vi "GenerateCmd.vi"(7 "Cmd":T1, 8 "error in":errorcluster, 10 "exp#":string, 11 "lang.font.exp":string) -> (0 "error Out":errorcluster, 3 "CMD":string)   [LabVIEW 2019]
uses:
  Controls/cmd.ctl
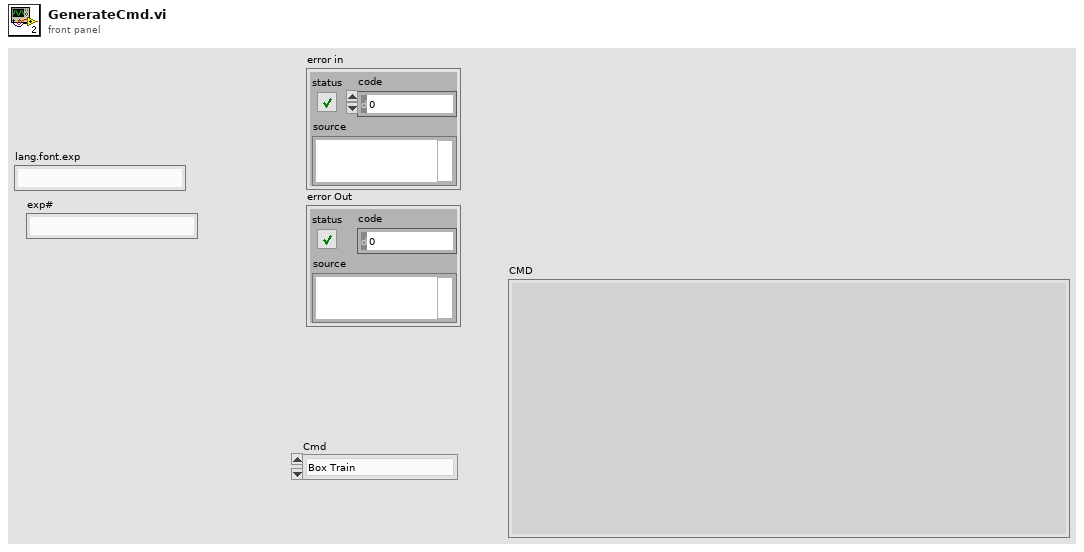
[diagram p1: front panel]
types:
  T1 = typedef "cmd.ctl" = enum16{"Box Train", "unicharset", "ShapeTable", "mftraining1", "mftraining2", "cntraining", "rename", "move files", "combine"}
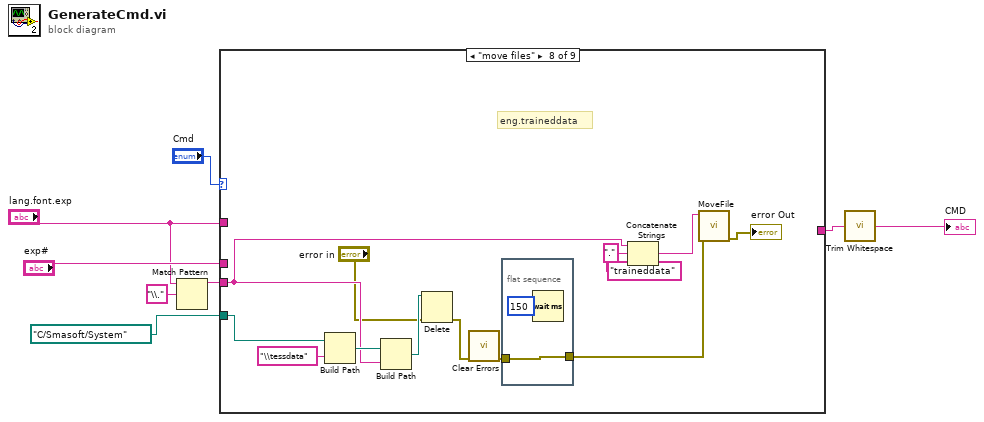
[diagram p0: block diagram]
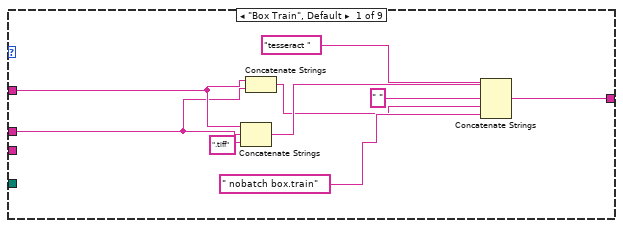
[diagram p2: hidden frame]
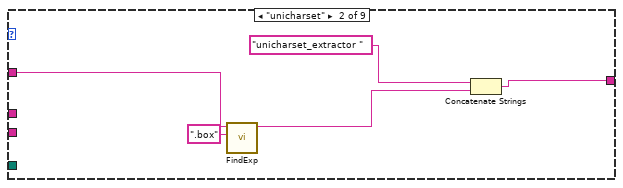
[diagram p3: hidden frame]
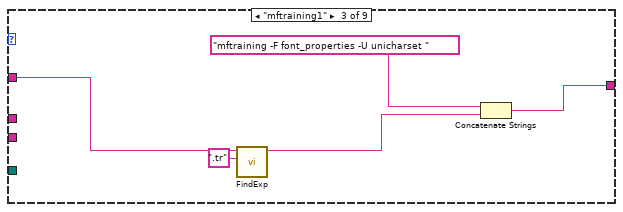
[diagram p4: hidden frame]
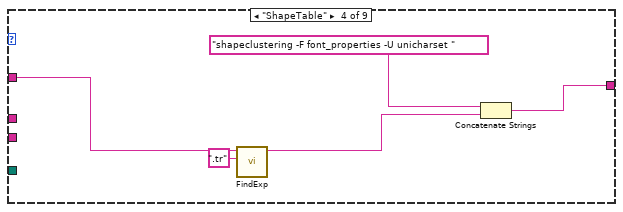
[diagram p5: hidden frame]
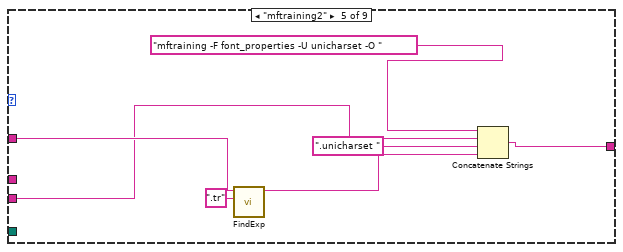
[diagram p6: hidden frame]
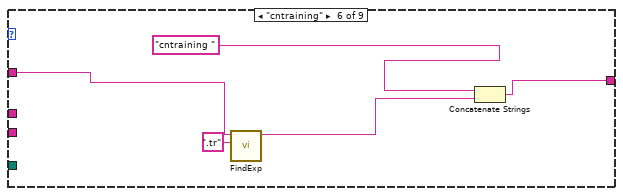
[diagram p7: hidden frame]
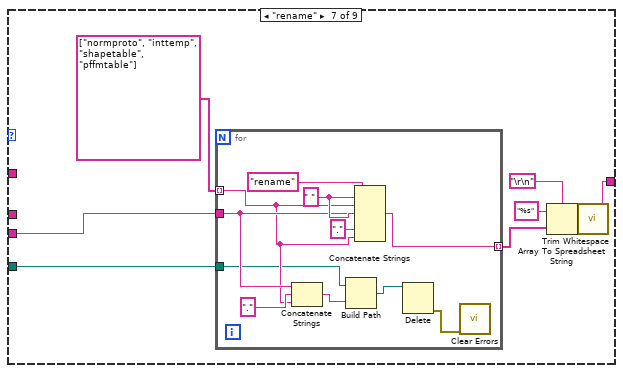
[diagram p8: hidden frame]
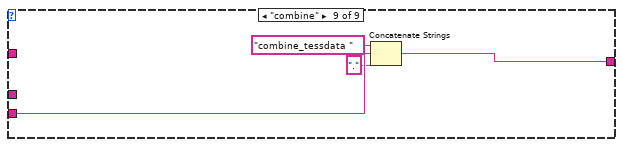
[diagram p9: hidden frame]
diagram:
  n1 = Match Pattern(string="lang.font.exp", regular expression="\\.") -> (before substring=w4:string)  [unwired: 1 in, 3 out]
  n2 = case shown="\"move files\"" "Cmd" {
    tunnel: "lang.font.exp" -> [w11 w20 w25 w30 w37 w41 _ _ _]
    tunnel: [w16 w22 w23 w28 w36 w40 w46 _ w79] -> w3
    tunnel: "exp#" -> [w10 _ _ _ _ _ _ _ _]
    tunnel: w4 -> [_ _ _ _ w34 _ w52 w69 w81]
    tunnel: path "C:/Smasoft/System" ("base path") -> [_ _ _ _ _ _ w45 w72 _]
    frame "Box Train", Default {
      n3 = Concatenate Strings(w11, w10, ".tiff" ("lang.font.exp")) -> (w15:string)
      n4 = Concatenate Strings(w11, w10) -> (w9:string)
      n5 = Concatenate Strings("tesseract ", w15, " " ("string"), w9, " nobatch box.train" ("string")) -> (w16:string)
    }
    frame "unicharset" {
      n6 = call "FindExp.vi"("extension name"=".box", "lang_font.exp"=w20) -> ("spreadsheet string"=w19:string)  [unwired: 9 in]
      n7 = Concatenate Strings("unicharset_extractor ", w19) -> (w22:string)
    }
    frame "mftraining1" {
      n8 = call "FindExp.vi"("extension name"=".tr", "lang_font.exp"=w25) -> ("spreadsheet string"=w26:string)  [unwired: 9 in]
      n9 = Concatenate Strings("mftraining -F font_properties -U unicharset ", w26) -> (w23:string)
    }
    frame "ShapeTable" {
      n10 = call "FindExp.vi"("extension name"=".tr", "lang_font.exp"=w30) -> ("spreadsheet string"=w31:string)  [unwired: 9 in]
      n11 = Concatenate Strings("shapeclustering -F font_properties -U unicharset ", w31) -> (w28:string)
    }
    frame "mftraining2" {
      n12 = call "FindExp.vi"("extension name"=".tr", "lang_font.exp"=w37) -> ("spreadsheet string"=w38:string)  [unwired: 9 in]
      n13 = Concatenate Strings("mftraining -F font_properties -U unicharset -O ", w34, ".unicharset " ("string"), w38) -> (w36:string)
    }
    frame "cntraining" {
      n14 = call "FindExp.vi"("extension name"=".tr", "lang_font.exp"=w41) -> ("spreadsheet string"=w42:string)  [unwired: 9 in]
      n15 = Concatenate Strings("cntraining ", w42) -> (w40:string)
    }
    frame "rename" {
      n16 = for {
        tunnel: string[] ["normproto", "inttemp", "shapetable", "pffmtable"] ("File name") -> [w57] mode=indexing
        tunnel: w52 -> [w59]
        tunnel: [w60] -> w50 mode=indexing
        tunnel: w45 -> [w55]
        w62 = " " ("string")
        n17 = Concatenate Strings(w59, "." ("string"), w57) -> (w56:string)
        n18 = Build Path(base path=w55, name or relative path=w56) -> (appended path=w54:path)
        n19 = Concatenate Strings("rename" ("string"), w62, w57, w62, w59, "." ("string"), w57) -> (w60:string)
        n20 = Delete(path (use dialog)=w54) -> (error out=w53:errorcluster)  [unwired: 4 in, 2 out]
        n21 = call <vilib>:"Clear Errors.vi"("error in (no error)"=w53) -> ()  [unwired: 5 in, 2 out]
      }
      n22 = Array To Spreadsheet String(delimiter (Tab)="\r\n", array=w50, 3:"%s" ("format string")) -> (spreadsheet string=w47:string)
      n23 = call <vilib>:"Trim Whitespace.vi"("string"=w47) -> ("trimmed string"=w46:string)  [unwired: 1 in]
    }
    frame "move files" {
      # "eng.traineddata"
      n24 = Build Path(base path=w72, name or relative path="\\tessdata") -> (appended path=w70:path)
      n25 = Build Path(base path=w70, name or relative path=w69) -> (appended path=w68:path)
      n26 = Delete(path (use dialog)=w68, error in="error in") -> (error out=w67:errorcluster)  [unwired: 3 in, 2 out]
      n27 = call <vilib>:"Clear Errors.vi"("error in (no error)"=w67) -> ("error out"=w65:errorcluster)  [unwired: 5 in, 1 out]
      n28 = flat-sequence {
        tunnel: [w78] -> w66
        tunnel: w65 -> [w78]
        frame #0 {
          n29 = Wait (ms)(milliseconds to wait=u32 150) -> ()  [unwired: 1 out]
        }
      }
      n30 = Concatenate Strings(w69, "." ("string"), "traineddata" ("string")) -> (w74:string)
      n31 = call "MoveFile.vi"("error in"=w66, "File Name"=w74) -> ("error out"=→"error Out":errorcluster)  [unwired: 9 in]
    }
    frame "combine" {
      n32 = Concatenate Strings("combine_tessdata " ("string"), w81, "." ("string")) -> (w79:string)
    }
  }
  n33 = call <vilib>:"Trim Whitespace.vi"("string"=w3) -> ("trimmed string"=→"CMD":string)  [unwired: 1 in]
